vi "SP Convert Display Cluster.vi"(4 "Conversion":enum16{"Cluster - HTML", "HTML - Cluster"}(ring), 6 "Display Key Array In":T9, 7 "Display Cluster In":T1={"Lock Control"=FALSE, "Retain Settings"=TRUE, "Formatted Data"=FALSE, "Plot Orientation"=enum."Single", "Plot Controls"=[{"Trace Orientation"=enum."Overlay", "Frequency"={"Change Frequency"=FALSE, "Start"=500.0, "Stop"=1500.0, "Units"=enum."MHz"}, "Markers"=[], "Traces"=[]}, {"Trace Orientation"=enum."Overlay", "Frequency"={"Change Frequency"=FALSE, "Start"=500.0, "Stop"=1500.0, "Units"=enum."MHz"}, "Markers"=[], "Traces"=[]}, {"Trace Orientation"=enum."Overlay", "Frequency"={"Change Frequency"=FALSE, "Start"=500.0, "Stop"=1500.0, "Units"=enum."MHz"}, "Markers"=[], "Traces"=[]}, {"Trace Orientation"=enum."Overlay", "Frequency"={"Change Frequency"=FALSE, "Start"=500.0, "Stop"=1500.0, "Units"=enum."MHz"}, "Markers"=[], "Traces"=[]}]} {"Plot Controls"."Traces"."Reference" format="%#.2g"; "Plot Controls"."Traces"."Display Data" items=["Data", "Memory", "Data/Memory"]; "Plot Controls"."Traces"."Format" items=["Log Mag", "Phase", "Expanded Phase", "Delay", "Smith", "Polar", "Lin Mag", "SWR", "Loss", "Real", "Imaginary"]; "Plot Controls"."Traces"."Scale" min=0.001 step=1.0 format="%#.2g"; "Plot Controls"."Traces"."Position" min=0.0 max=10.0; "Plot Controls"."Frequency"."Stop" format="%.3g"; "Plot Controls"."Frequency"."Start" format="%.3g"}) -> (1 "Display Cluster Out":T1={"Lock Control"=FALSE, "Retain Settings"=TRUE, "Formatted Data"=FALSE, "Plot Orientation"=enum."Single", "Plot Controls"=[{"Trace Orientation"=enum."Overlay", "Frequency"={"Change Frequency"=FALSE, "Start"=500.0, "Stop"=1500.0, "Units"=enum."MHz"}, "Markers"=[], "Traces"=[]}, {"Trace Orientation"=enum."Overlay", "Frequency"={"Change Frequency"=FALSE, "Start"=500.0, "Stop"=1500.0, "Units"=enum."MHz"}, "Markers"=[], "Traces"=[]}, {"Trace Orientation"=enum."Overlay", "Frequency"={"Change Frequency"=FALSE, "Start"=500.0, "Stop"=1500.0, "Units"=enum."MHz"}, "Markers"=[], "Traces"=[]}, {"Trace Orientation"=enum."Overlay", "Frequency"={"Change Frequency"=FALSE, "Start"=500.0, "Stop"=1500.0, "Units"=enum."MHz"}, "Markers"=[], "Traces"=[]}]} {"Plot Controls"."Traces"."Reference" format="%#.2g"; "Plot Controls"."Traces"."Display Data" items=["Data", "Memory", "Data/Memory"]; "Plot Controls"."Traces"."Format" items=["Log Mag", "Phase", "Expanded Phase", "Delay", "Smith", "Polar", "Lin Mag", "SWR", "Loss", "Real", "Imaginary"]; "Plot Controls"."Traces"."Scale" min=0.001 step=1.0 format="%#.2g"; "Plot Controls"."Traces"."Position" min=0.0 max=10.0; "Plot Controls"."Frequency"."Stop" format="%.3g"; "Plot Controls"."Frequency"."Start" format="%.3g"}, 2 "Display HTML Out":string)   [LabVIEW 2011]
uses:
  ITK/utils/keyedarr.llb/Keyed Array.ctl
  TypeDefs/SP Display Parameters.ctl
  TypeDefs/SP Display Plot Controls Cluster.ctl
  TypeDefs/SP Frequency Units.ctl
  TypeDefs/SP Marker Cluster.ctl
  TypeDefs/SP Marker Type.ctl
  TypeDefs/SP Display Trace Controls.ctl
  TypeDefs/SP Display Format.ctl
  TypeDefs/SP Display Data.ctl
  ITK/utils/strutil.llb/Case Matching.ctl
panel:
  # "Div"
  # "Div"
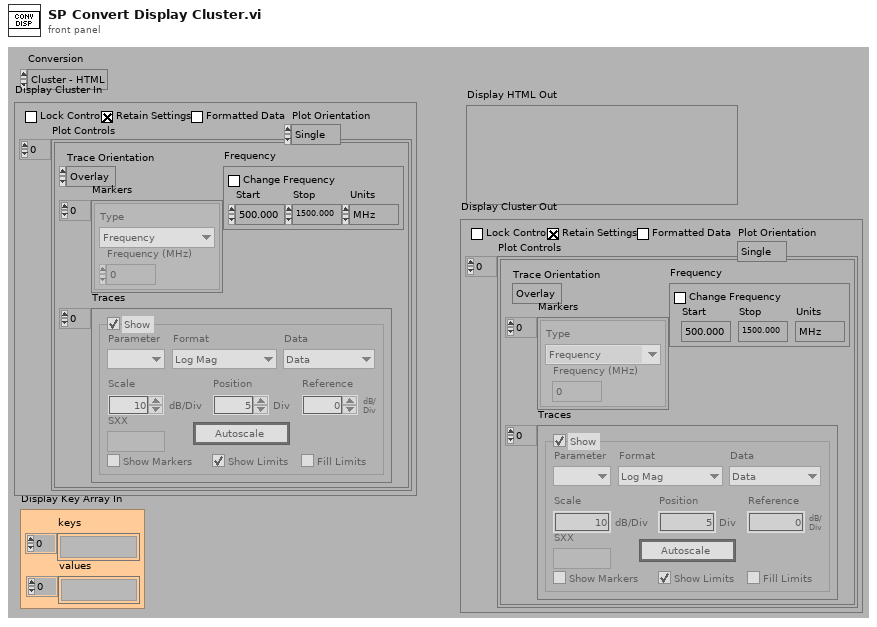
[diagram p1: front panel]
types:
  T1 = typedef "SP Display Parameters.ctl" = cluster{"Lock Control":bool, "Retain Settings":bool, "Formatted Data":bool, "Plot Orientation":enum32{"Single", "Dual", "Quad"}, "Plot Controls":T2[]}
  T2 = typedef "SP Display Plot Controls Cluster.ctl" = cluster{"Trace Orientation":enum32{"Overlay", "Split"}, "Frequency":cluster{"Change Frequency":bool, "Start":dbl, "Stop":dbl, "Units":T3}, "Markers":T4[], "Traces":T6[]}
  T3 = typedef "SP Frequency Units.ctl" = enum16{"Hz", "kHz", "MHz", "GHz", "Points"}
  T4 = typedef "SP Marker Cluster.ctl" = cluster{"Type":T5, "Frequency (MHz)":dbl}
  T5 = typedef "SP Marker Type.ctl" = enum16{"Frequency", "Trace Maximum", "Trace Minimum", "Limit Maximum", "Limit Minimum"}
  T6 = typedef "SP Display Trace Controls.ctl" = cluster{"Trace On":bool, "Measure":i32, "Format":T7, "Autoscale":bool, "Reference":dbl, "\nRefUnit":string, "Position":dbl, "Scale":dbl, "ScaleUnit":string, "LimitOn":bool, "LimitFill":bool, "Display Data":T8, "Show Markers":bool, "SXX":string}
  T7 = typedef "SP Display Format.ctl" = i32
  T8 = typedef "SP Display Data.ctl" = u16
  T9 = typedef "Keyed Array.ctl" = cluster{"keys":string[], "values":string[]}
  T10 = typedef "SP Parameter.ctl" = cluster{"Stimulus Port":i8, "Response Port":i8}
  T11 = typedef "Case Matching.ctl" = enum16{"a != A", "a == A", "system"}
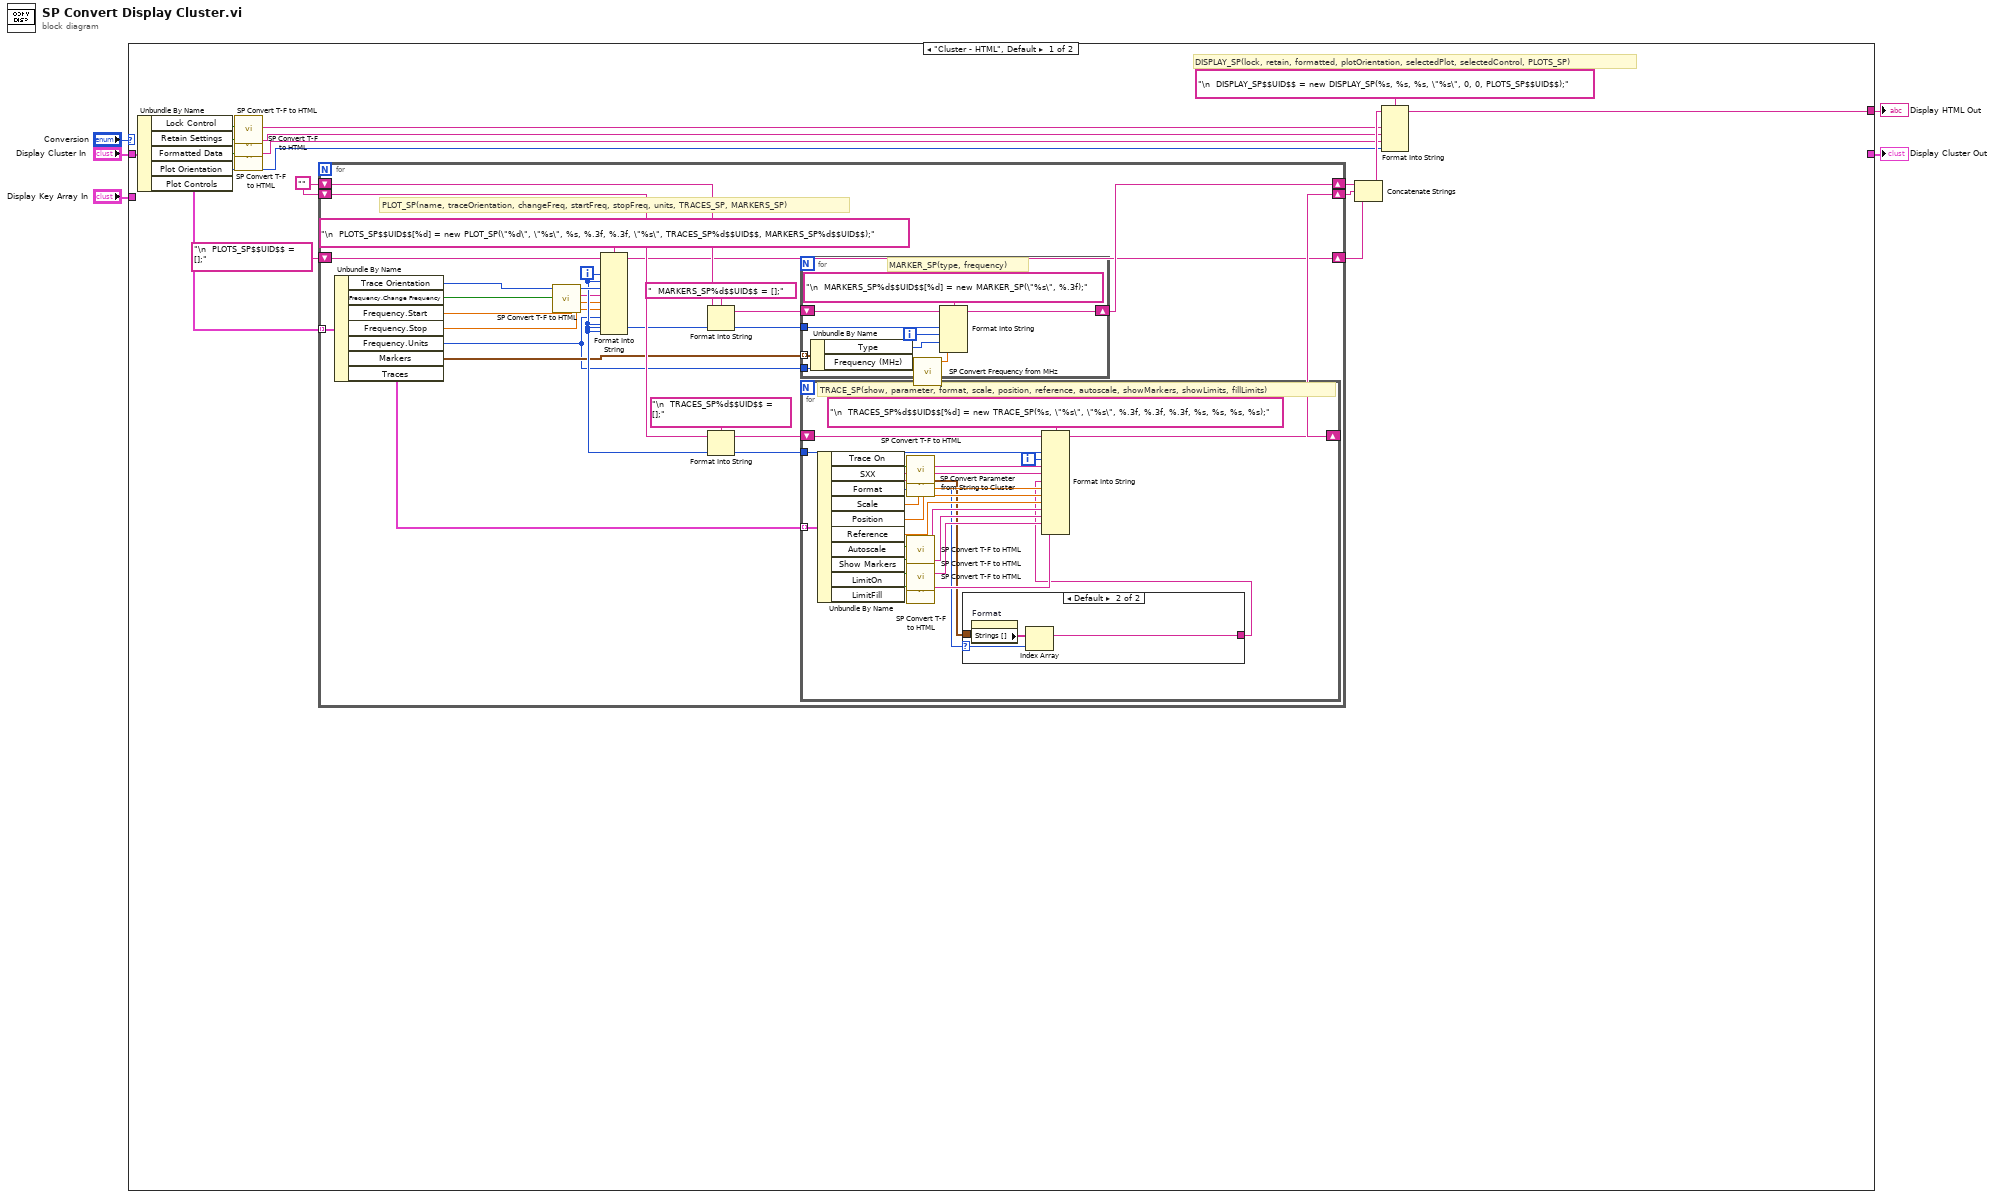
[diagram p0: block diagram]
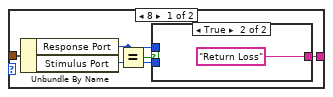
[diagram p2: hidden frame]
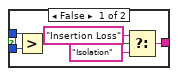
[diagram p3: hidden frame]
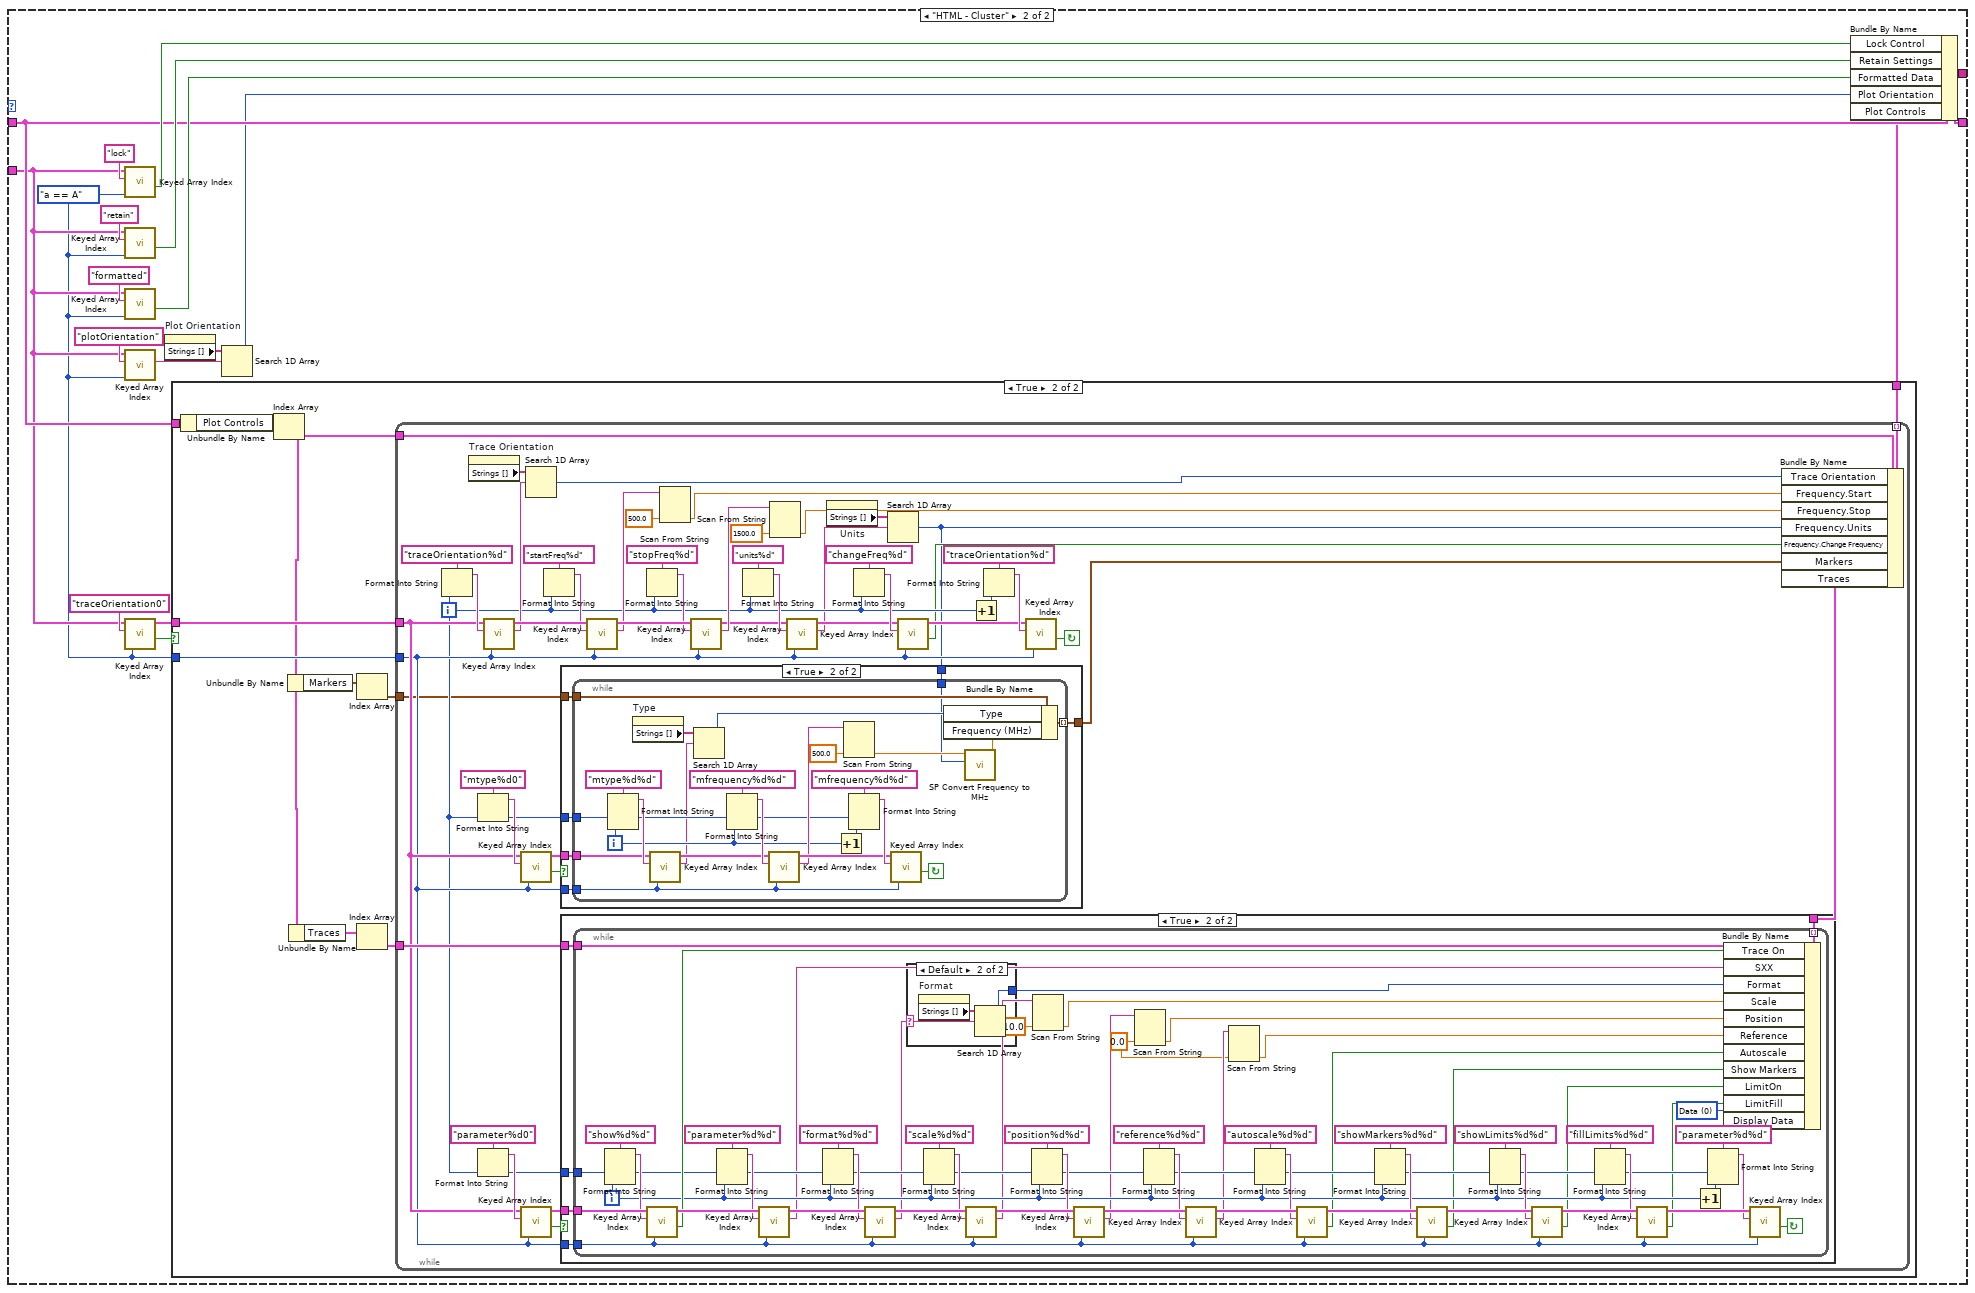
[diagram p4: hidden frame]
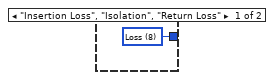
[diagram p7: hidden frame]
diagram:
  n1 = case shown="\"Cluster - HTML\", Default" "Conversion" {
    tunnel: "Display Cluster In" -> [w13 w102]
    tunnel: "Display Key Array In" -> [_ w95]
    tunnel: [w12 _] -> w2
    tunnel: [_ w97] -> w1
    frame "Cluster - HTML", Default {
      w8 = ""
      # "DISPLAY_SP(lock, retain, formatted, plotOrientation, selectedPlot, selectedControl, PLOTS_SP)"
      n2 = Unbundle By Name(w13) -> ("Lock Control"=w15:bool, "Retain Settings"=w18:bool, "Formatted Data"=w17:bool, "Plot Orientation"=w21:enum32{"Single", "Dual", "Quad"}, "Plot Controls"=w11:T2[])
      n3 = call "SP Convert T-F to HTML.vi"("(T/F)"=w15) -> ("HTML (true/false)"=w16:string)  [unwired: 10 out]
      n4 = call "SP Convert T-F to HTML.vi"("(T/F)"=w18) -> ("HTML (true/false)"=w19:string)  [unwired: 10 out]
      n5 = call "SP Convert T-F to HTML.vi"("(T/F)"=w17) -> ("HTML (true/false)"=w20:string)  [unwired: 10 out]
      n6 = for {
        tunnel: w11 -> [w43] mode=indexing
        shift-right: [w30] -> w9
        shift-left: "\n  PLOTS_SP$$UID$$ = [];" ("format string") -> [w42]
        shift-right: [w34] -> w7
        shift-left: w8 -> [w35]
        shift-right: [w33] -> w6
        shift-left: w8 -> [w32]
        i -> [w29]
        # "PLOT_SP(name, traceOrientation, changeFreq, startFreq, stopFreq, units, TRACES_SP, MARKERS_SP)"
        n7 = Unbundle By Name(w43) -> ("Trace Orientation"=w41:enum32{"Overlay", "Split"}, "Frequency.Change Frequency"=w25:bool, "Frequency.Start"=w28:dbl, "Frequency.Stop"=w27:dbl, "Frequency.Units"=w23:T3, "Markers"=w24:T4[], "Traces"=w31:T6[])
        n8 = call "SP Convert T-F to HTML.vi"("(T/F)"=w25) -> ("HTML (true/false)"=w26:string)  [unwired: 10 out]
        n9 = Format Into String(format string="\n  PLOTS_SP$$UID$$[%d] = new PLOT_SP(\"%d\", \"%s\", %s, %.3f, %.3f, \"%s\", TRACES_SP%d$$UID$$, MARKERS_SP%d$$UID$$);", initial string=w42, w29, w29, w41, w26, w28, w27, w23, w29, w29) -> (resulting string=w30:string)  [unwired: 1 in, 1 out]
        n10 = Format Into String(format string="  MARKERS_SP%d$$UID$$ = [];", initial string=w35, w29) -> (resulting string=w38:string)  [unwired: 1 in, 1 out]
        n11 = Format Into String(format string="\n  TRACES_SP%d$$UID$$ = [];", initial string=w32, w29) -> (resulting string=w37:string)  [unwired: 1 in, 1 out]
        n12 = for {
          tunnel: w24 -> [w86] mode=indexing
          shift-right: [w89] -> w34
          shift-left: w38 -> [w90]
          tunnel: w29 -> [w87]
          tunnel: w23 -> [w82]
          i -> [w88]
          # "MARKER_SP(type, frequency)"
          n13 = Unbundle By Name(w86) -> ("Type"=w85:T5, "Frequency (MHz)"=w84:dbl)
          n14 = call "SP Convert Frequency from MHz.vi"("Units"=w82, "Frequency (MHz)"=w84) -> ("Converted Frequency"=w83:dbl)  [unwired: 1 in, 8 out]
          n15 = Format Into String(format string="\n  MARKERS_SP%d$$UID$$[%d] = new MARKER_SP(\"%s\", %.3f);", initial string=w90, w87, w88, w85, w83) -> (resulting string=w89:string)  [unwired: 1 in, 1 out]
        }
        n16 = for {
          tunnel: w31 -> [w63] mode=indexing
          shift-right: [w64] -> w33
          shift-left: w37 -> [w65]
          tunnel: w29 -> [w48]
          i -> [w49]
          # "TRACE_SP(show, parameter, format, scale, position, reference, autoscale, showMarkers, showLimits, fillLimits)"
          n17 = Unbundle By Name(w63) -> ("Trace On"=w62:bool, "SXX"=w47:string, "Format"=w46:T7, "Scale"=w60:dbl, "Position"=w59:dbl, "Reference"=w58:dbl, "Autoscale"=w57:bool, "Show Markers"=w54:bool, "LimitOn"=w55:bool, "LimitFill"=w56:bool)
          n18 = call "SP Convert T-F to HTML.vi"("(T/F)"=w62) -> ("HTML (true/false)"=w61:string)  [unwired: 10 out]
          n19 = call "SP Convert Parameter from String to Cluster.vi"("Parameter String"=w47) -> ("Parameter"=w45:T10)  [unwired: 10 out]
          n20 = call "SP Convert T-F to HTML.vi"("(T/F)"=w57) -> ("HTML (true/false)"=w53:string)  [unwired: 10 out]
          n21 = call "SP Convert T-F to HTML.vi"("(T/F)"=w54) -> ("HTML (true/false)"=w52:string)  [unwired: 10 out]
          n22 = call "SP Convert T-F to HTML.vi"("(T/F)"=w55) -> ("HTML (true/false)"=w51:string)  [unwired: 10 out]
          n23 = call "SP Convert T-F to HTML.vi"("(T/F)"=w56) -> ("HTML (true/false)"=w50:string)  [unwired: 10 out]
          n24 = case shown="Default" w46 {
            selector: w46 -> [_ w80]
            tunnel: w45 -> [w71 _]
            tunnel: [w67 w79] -> w44
            frame 8 {
              n25 = Unbundle By Name(w71) -> ("Response Port"=w69:i8, "Stimulus Port"=w68:i8)
              n26 = Equal?(x=w69, y=w68) -> (x = y?=w70:bool)
              n27 = case shown="True" w70 {
                tunnel: [w74 "Return Loss" ("format string")] -> w67
                tunnel: w69 -> [w77 _]
                tunnel: w68 -> [w76 _]
                frame False {
                  n28 = Greater?(x=w77, y=w76) -> (0:w75:bool)
                  n29 = Select(t="Insertion Loss" ("format string"), s=w75, f="Isolation" ("format string")) -> (s? t:f=w74:string)
                }
                frame True {
                }
              }
            }
            frame Default {
              n30 = property on="Format" class="Ring (strict)"() -> ("Strings []"=w81:string[])  [unwired: 2 in, 2 out]
              n31 = Index Array(array=w81, index=w80) -> (element=w79:string)
            }
          }
          n32 = Format Into String(format string="\n  TRACES_SP%d$$UID$$[%d] = new TRACE_SP(%s, \"%s\", \"%s\", %.3f, %.3f, %.3f, %s, %s, %s, %s);", initial string=w65, w48, w49, w61, w47, w44, w60, w59, w58, w53, w52, w51, w50) -> (resulting string=w64:string)  [unwired: 1 in, 1 out]
        }
      }
      n33 = Concatenate Strings(w7, w6, w9) -> (w22:string)
      n34 = Format Into String(format string="\n  DISPLAY_SP$$UID$$ = new DISPLAY_SP(%s, %s, %s, \"%s\", 0, 0, PLOTS_SP$$UID$$);", initial string=w22, w16, w19, w20, w21) -> (resulting string=w12:string)  [unwired: 1 in, 1 out]
    }
    frame "HTML - Cluster" {
      w93 = Case_Matching."a == A" ("case matching (sensitive)")
      n35 = call "Keyed Array Index.vi"("case matching (sensitive)"=w93, "key"="lock", "array in"=w95) -> ("valid key"=w107:bool)  [unwired: 1 in, 3 out]
      n36 = call "Keyed Array Index.vi"("case matching (sensitive)"=w93, "key"="retain", "array in"=w95) -> ("valid key"=w108:bool)  [unwired: 1 in, 3 out]
      n37 = call "Keyed Array Index.vi"("case matching (sensitive)"=w93, "key"="formatted", "array in"=w95) -> ("valid key"=w103:bool)  [unwired: 1 in, 3 out]
      n38 = call "Keyed Array Index.vi"("case matching (sensitive)"=w93, "key"="plotOrientation", "array in"=w95) -> ("value"=w101:string)  [unwired: 1 in, 3 out]
      n39 = call "Keyed Array Index.vi"("case matching (sensitive)"=w93, "key"="traceOrientation0", "array in"=w95) -> ("valid key"=w92:bool, "duplicate array"=w94:T9)  [unwired: 1 in, 2 out]
      n40 = property on="Plot Orientation" class="Enum (strict)"() -> ("Strings []"=w100:string[])  [unwired: 2 in, 2 out]
      n41 = case shown="True" w92 {
        tunnel: w102 -> [_ w118]
        tunnel: [_ w115] -> w98
        tunnel: w94 -> [_ w114]
        tunnel: w93 -> [_ w113]
        frame False {
        }
        frame True {
          n42 = Unbundle By Name(w118) -> ("Plot Controls"=w119:T2[])
          n43 = Index Array(array=w119) -> (element=w112:T2)  [unwired: 1 in]
          n44 = Unbundle By Name(w112) -> ("Markers"=w111:T4[])
          n45 = Unbundle By Name(w112) -> ("Traces"=w117:T6[])
          n46 = Index Array(array=w111) -> (element=w110:T4)  [unwired: 1 in]
          n47 = Index Array(array=w117) -> (element=w116:T6)  [unwired: 1 in]
          n48 = while {
            tunnel: w112 -> [w166]
            tunnel: w113 -> [w130]
            tunnel: w114 -> [w137]
            tunnel: w116 -> [w146]
            tunnel: [w144] -> w115 mode=indexing
            tunnel: w110 -> [w121]
            i -> [w126]
            stop <- w154 continue-if-true
            n49 = Format Into String(format string="traceOrientation%d", w126) -> (resulting string=w164:string)  [unwired: 2 in, 1 out]
            n50 = property on="Trace Orientation" class="Enum (strict)"() -> ("Strings []"=w151:string[])  [unwired: 2 in, 2 out]
            n51 = Format Into String(format string="mtype%d0", w126) -> (resulting string=w140:string)  [unwired: 2 in, 1 out]
            n52 = Format Into String(format string="parameter%d0", w126) -> (resulting string=w139:string)  [unwired: 2 in, 1 out]
            n53 = call "Keyed Array Index.vi"("case matching (sensitive)"=w130, "key"=w164, "array in"=w137) -> ("value"=w150:string, "duplicate array"=w167:T9)  [unwired: 1 in, 2 out]
            n54 = call "Keyed Array Index.vi"("case matching (sensitive)"=w130, "key"=w140, "array in"=w137) -> ("valid key"=w143:bool, "duplicate array"=w142:T9)  [unwired: 1 in, 2 out]
            n55 = call "Keyed Array Index.vi"("case matching (sensitive)"=w130, "key"=w139, "array in"=w137) -> ("valid key"=w135:bool, "duplicate array"=w136:T9)  [unwired: 1 in, 2 out]
            n56 = Search 1D Array(1D array=w151, element=w150) -> (index of element=w149:i32)  [unwired: 1 out]
            n57 = Format Into String(format string="startFreq%d", w126) -> (resulting string=w161:string)  [unwired: 2 in, 1 out]
            n58 = case shown="True" w135 {
              tunnel: w146 -> [_ w173]
              tunnel: [_ w172] -> w145
              tunnel: w136 -> [_ w171]
              tunnel: w130 -> [_ w170]
              tunnel: w126 -> [_ w169]
              frame False {
              }
              frame True {
                n59 = while {
                  tunnel: w171 -> [w230]
                  tunnel: w170 -> [w190]
                  tunnel: w173 -> [w213]
                  tunnel: w169 -> [w191]
                  tunnel: [w175] -> w172 mode=indexing
                  i -> [w192]
                  stop <- w214 continue-if-true
                  w180 = 0.0 ("default value 1")
                  w212 = T8 0 items=["Data", "Memory", "Data/Memory"] ("Display Data")
                  n60 = Format Into String(format string="show%d%d", w191, w192) -> (resulting string=w219:string)  [unwired: 2 in, 1 out]
                  n61 = call "Keyed Array Index.vi"("case matching (sensitive)"=w190, "key"=w219, "array in"=w230) -> ("valid key"=w211:bool, "duplicate array"=w229:T9)  [unwired: 1 in, 2 out]
                  n62 = Format Into String(format string="parameter%d%d", w191, w192) -> (resulting string=w209:string)  [unwired: 2 in, 1 out]
                  n63 = call "Keyed Array Index.vi"("case matching (sensitive)"=w190, "key"=w209, "array in"=w229) -> ("value"=w189:string, "duplicate array"=w228:T9)  [unwired: 1 in, 2 out]
                  n64 = Format Into String(format string="format%d%d", w191, w192) -> (resulting string=w208:string)  [unwired: 2 in, 1 out]
                  n65 = call "Keyed Array Index.vi"("case matching (sensitive)"=w190, "key"=w208, "array in"=w228) -> ("value"=w174:string, "duplicate array"=w227:T9)  [unwired: 1 in, 2 out]
                  n66 = case shown="Default" w174 {
                    selector: w174 -> [_ w232]
                    tunnel: [w231 w233] -> w188
                    frame "Insertion Loss", "Isolation", "Return Loss" {
                      w231 = T7 8 items=["Log Mag", "Phase", "Expanded Phase", "Delay", "Smith", "Polar", "Lin Mag", "SWR", "Loss", "Real", "Imaginary"] ("Format")
                    }
                    frame Default {
                      n67 = property on="Format" class="Ring (strict)"() -> ("Strings []"=w234:string[])  [unwired: 2 in, 2 out]
                      n68 = Search 1D Array(1D array=w234, element=w232) -> (index of element=w233:i32)  [unwired: 1 out]
                    }
                  }
                  n69 = Format Into String(format string="scale%d%d", w191, w192) -> (resulting string=w205:string)  [unwired: 2 in, 1 out]
                  n70 = call "Keyed Array Index.vi"("case matching (sensitive)"=w190, "key"=w205, "array in"=w227) -> ("value"=w186:string, "duplicate array"=w226:T9)  [unwired: 1 in, 2 out]
                  n71 = Format Into String(format string="position%d%d", w191, w192) -> (resulting string=w204:string)  [unwired: 2 in, 1 out]
                  n72 = Scan From String(input string=w186, default 1=10.0 ("default value 1")) -> (output 1=w185:dbl)  [unwired: 3 in, 3 out]
                  n73 = call "Keyed Array Index.vi"("case matching (sensitive)"=w190, "key"=w204, "array in"=w226) -> ("value"=w184:string, "duplicate array"=w225:T9)  [unwired: 1 in, 2 out]
                  n74 = Scan From String(input string=w184, default 1=w180) -> (output 1=w183:dbl)  [unwired: 3 in, 3 out]
                  n75 = Format Into String(format string="reference%d%d", w191, w192) -> (resulting string=w201:string)  [unwired: 2 in, 1 out]
                  n76 = call "Keyed Array Index.vi"("case matching (sensitive)"=w190, "key"=w201, "array in"=w225) -> ("value"=w182:string, "duplicate array"=w224:T9)  [unwired: 1 in, 2 out]
                  n77 = Scan From String(input string=w182, default 1=w180) -> (output 1=w181:dbl)  [unwired: 3 in, 3 out]
                  n78 = Format Into String(format string="autoscale%d%d", w191, w192) -> (resulting string=w200:string)  [unwired: 2 in, 1 out]
                  n79 = call "Keyed Array Index.vi"("case matching (sensitive)"=w190, "key"=w200, "array in"=w224) -> ("valid key"=w179:bool, "duplicate array"=w223:T9)  [unwired: 1 in, 2 out]
                  n80 = Format Into String(format string="showMarkers%d%d", w191, w192) -> (resulting string=w197:string)  [unwired: 2 in, 1 out]
                  n81 = call "Keyed Array Index.vi"("case matching (sensitive)"=w190, "key"=w197, "array in"=w223) -> ("valid key"=w178:bool, "duplicate array"=w222:T9)  [unwired: 1 in, 2 out]
                  n82 = Format Into String(format string="showLimits%d%d", w191, w192) -> (resulting string=w196:string)  [unwired: 2 in, 1 out]
                  n83 = call "Keyed Array Index.vi"("case matching (sensitive)"=w190, "key"=w196, "array in"=w222) -> ("valid key"=w177:bool, "duplicate array"=w221:T9)  [unwired: 1 in, 2 out]
                  n84 = Format Into String(format string="fillLimits%d%d", w191, w192) -> (resulting string=w193:string)  [unwired: 2 in, 1 out]
                  n85 = call "Keyed Array Index.vi"("case matching (sensitive)"=w190, "key"=w193, "array in"=w221) -> ("valid key"=w176:bool, "duplicate array"=w220:T9)  [unwired: 1 in, 2 out]
                  n86 = Increment(x=w192) -> (x+1=w215:i32)
                  n87 = Format Into String(format string="parameter%d%d", w191, w215) -> (resulting string=w216:string)  [unwired: 2 in, 1 out]
                  n88 = Bundle By Name(cluster=w213, "Trace On"=w211, "SXX"=w189, "Format"=w188, "Scale"=w185, "Position"=w183, "Reference"=w181, "Autoscale"=w179, "Show Markers"=w178, "LimitOn"=w177, "LimitFill"=w176, "Display Data"=w212) -> (w175:T6)
                  n89 = call "Keyed Array Index.vi"("case matching (sensitive)"=w190, "key"=w216, "array in"=w220) -> ("valid key"=w214:bool)  [unwired: 1 in, 3 out]
                }
              }
            }
            n90 = call "Keyed Array Index.vi"("case matching (sensitive)"=w130, "key"=w161, "array in"=w167) -> ("value"=w159:string, "duplicate array"=w168:T9)  [unwired: 1 in, 2 out]
            n91 = Format Into String(format string="stopFreq%d", w126) -> (resulting string=w160:string)  [unwired: 2 in, 1 out]
            n92 = Scan From String(input string=w159, default 1=500.0 ("default value 1")) -> (output 1=w134:dbl)  [unwired: 3 in, 3 out]
            n93 = call "Keyed Array Index.vi"("case matching (sensitive)"=w130, "key"=w160, "array in"=w168) -> ("value"=w147:string, "duplicate array"=w129:T9)  [unwired: 1 in, 2 out]
            n94 = Format Into String(format string="units%d", w126) -> (resulting string=w152:string)  [unwired: 2 in, 1 out]
            n95 = Scan From String(input string=w147, default 1=1500.0 ("default value 1")) -> (output 1=w133:dbl)  [unwired: 3 in, 3 out]
            n96 = call "Keyed Array Index.vi"("case matching (sensitive)"=w130, "key"=w152, "array in"=w129) -> ("value"=w123:string, "duplicate array"=w128:T9)  [unwired: 1 in, 2 out]
            n97 = property on="Units" class="Enum (strict)"() -> ("Strings []"=w124:string[])  [unwired: 2 in, 2 out]
            n98 = Format Into String(format string="changeFreq%d", w126) -> (resulting string=w132:string)  [unwired: 2 in, 1 out]
            n99 = Search 1D Array(1D array=w124, element=w123) -> (index of element=w120:i32)  [unwired: 1 out]
            n100 = case shown="True" w143 {
              tunnel: [_ w240] -> w122
              tunnel: w130 -> [_ w239]
              tunnel: w142 -> [_ w238]
              tunnel: w126 -> [_ w237]
              tunnel: w121 -> [_ w236]
              tunnel: w120 -> [_ w235]
              frame False {
              }
              frame True {
                n101 = while {
                  tunnel: w238 -> [w251]
                  tunnel: w239 -> [w249]
                  tunnel: [w244] -> w240 mode=indexing
                  tunnel: w237 -> [w253]
                  tunnel: w236 -> [w245]
                  tunnel: w235 -> [w241]
                  i -> [w252]
                  stop <- w258 continue-if-true
                  n102 = Format Into String(format string="mtype%d%d", w253, w252) -> (resulting string=w254:string)  [unwired: 2 in, 1 out]
                  n103 = property on="Type" class="Enum (strict)"() -> ("Strings []"=w247:string[])  [unwired: 2 in, 2 out]
                  n104 = call "Keyed Array Index.vi"("case matching (sensitive)"=w249, "key"=w254, "array in"=w251) -> ("value"=w246:string, "duplicate array"=w250:T9)  [unwired: 1 in, 2 out]
                  n105 = Search 1D Array(1D array=w247, element=w246) -> (index of element=w242:i32)  [unwired: 1 out]
                  n106 = Format Into String(format string="mfrequency%d%d", w253, w252) -> (resulting string=w264:string)  [unwired: 2 in, 1 out]
                  n107 = call "Keyed Array Index.vi"("case matching (sensitive)"=w249, "key"=w264, "array in"=w250) -> ("value"=w256:string, "duplicate array"=w260:T9)  [unwired: 1 in, 2 out]
                  n108 = Increment(x=w252) -> (x+1=w259:i32)
                  n109 = Scan From String(input string=w256, default 1=500.0 ("default value 1")) -> (output 1=w248:dbl)  [unwired: 3 in, 3 out]
                  n110 = Format Into String(format string="mfrequency%d%d", w253, w259) -> (resulting string=w261:string)  [unwired: 2 in, 1 out]
                  n111 = call "Keyed Array Index.vi"("case matching (sensitive)"=w249, "key"=w261, "array in"=w260) -> ("valid key"=w258:bool)  [unwired: 1 in, 3 out]
                  n112 = call "SP Convert Frequency to MHz.vi"("Units"=w241, "Frequency"=w248) -> ("Converted Frequency"=w243:dbl)  [unwired: 1 in, 8 out]
                  n113 = Bundle By Name(cluster=w245, "Type"=w242, "Frequency (MHz)"=w243) -> (w244:T4)
                }
              }
            }
            n114 = call "Keyed Array Index.vi"("case matching (sensitive)"=w130, "key"=w132, "array in"=w128) -> ("valid key"=w125:bool, "duplicate array"=w127:T9)  [unwired: 1 in, 2 out]
            n115 = Increment(x=w126) -> (x+1=w156:i32)
            n116 = Format Into String(format string="traceOrientation%d", w156) -> (resulting string=w155:string)  [unwired: 2 in, 1 out]
            n117 = call "Keyed Array Index.vi"("case matching (sensitive)"=w130, "key"=w155, "array in"=w127) -> ("valid key"=w154:bool)  [unwired: 1 in, 3 out]
            n118 = Bundle By Name(cluster=w166, "Trace Orientation"=w149, "Frequency.Start"=w134, "Frequency.Stop"=w133, "Frequency.Units"=w120, "Frequency.Change Frequency"=w125, "Markers"=w122, "Traces"=w145) -> (w144:T2)
          }
        }
      }
      n119 = Search 1D Array(1D array=w100, element=w101) -> (index of element=w99:i32)  [unwired: 1 out]
      n120 = Bundle By Name(cluster=w102, "Lock Control"=w107, "Retain Settings"=w108, "Formatted Data"=w103, "Plot Orientation"=w99, "Plot Controls"=w98) -> (w97:T1)
    }
  }
  "Display HTML Out" <- w2
  "Display Cluster Out" <- w1
